vi "TDMS Write Telemtry Data.vi"(8 "error in (no error)":errorcluster, 11 "Iterations":i32) -> (0 "error out":errorcluster, 3 "TDMS file path":path)   [LabVIEW 2021]
doc: "This example demonstrates how to write measured data along with text and timestamp values to a .tdms file using the TDMS API. TDMS files written by this example can be read by the example TDMS Read Events Data.vi."
panel:
  in  "LogEvent":bool
  in  "Stop":bool
  out "Time Stamp":timestamp
  out "Description":string="Event XYZ"
  out "Measured Data":waveform(dbl)[](graph)
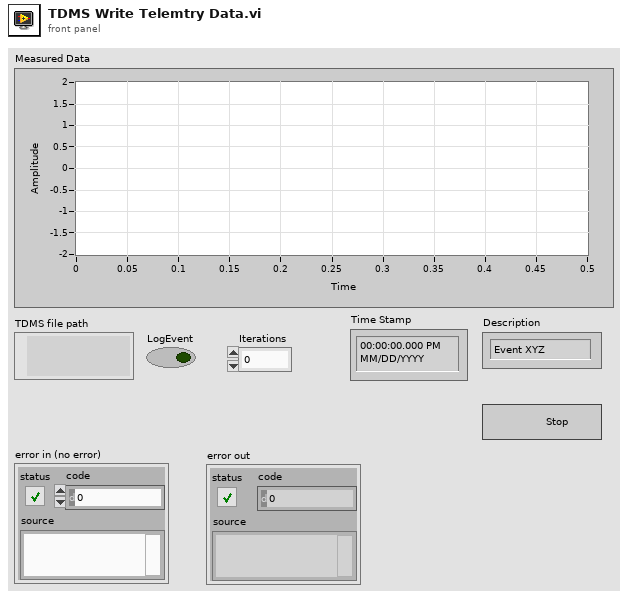
[diagram p1: front panel]
types:
  T1 = enum16{"open", "open or create", "create or replace", "create", "open (read-only)"}
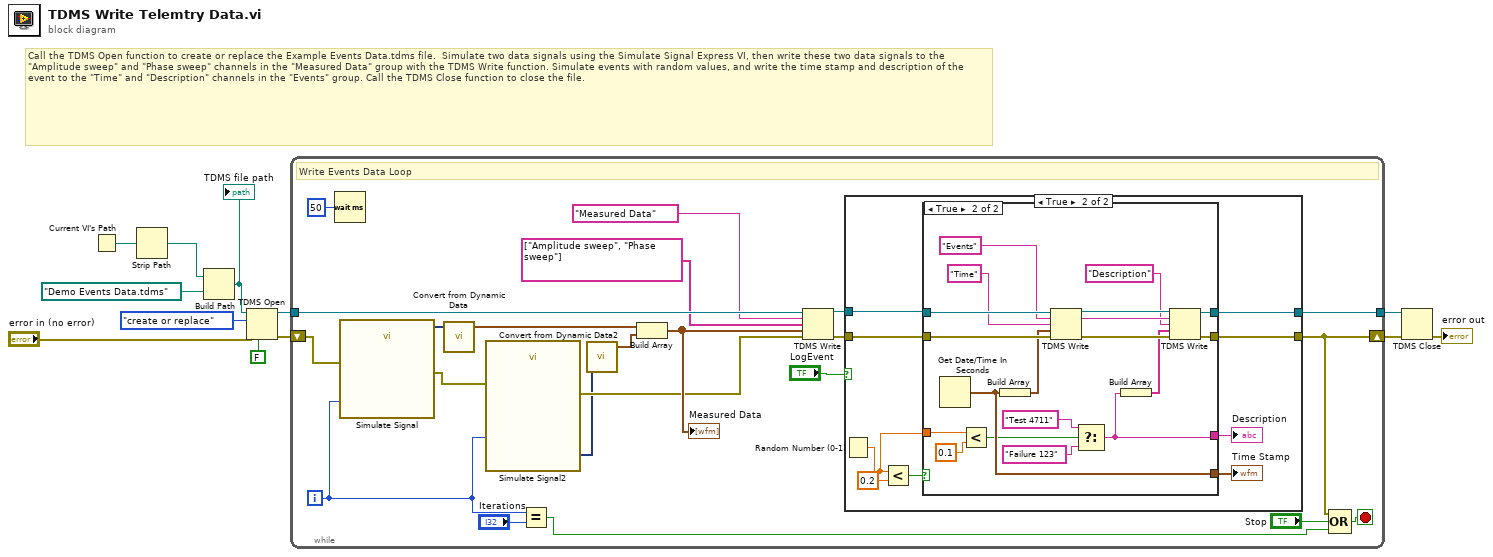
[diagram p0: block diagram]
diagram:
  # "Call the TDMS Open function to create or replace the Example Events Data.tdms file.  Simulate two data signals using the Simulate Signal Express VI, then write these two data signals to the \"Amplitude sweep\" and \"Phase sweep\" channels in the \"Measured Data\" group with the TDMS Write function. Simulate events with random values, and write the time stamp and description of the event to the \"Time\" and \"Description\" channels in the \"Events\" group. Call the TDMS Close function to close the file."
  n1 = Current VI's Path() -> (path=w12:path)
  n2 = Strip Path(path=w12) -> (stripped path=w1:path)  [unwired: 1 out]
  n3 = Build Path(base path=w1, name or relative path=path "Demo Events Data.tdms" ("file path")) -> (appended path=w5:path)
  "TDMS file path" <- w5
  n4 = TDMS Open(6:FALSE ("disable buffering (T)"), 8:"error in (no error)", 10:T1."create or replace" ("operation"), 11:w5) -> (0:w8:errorcluster, 3:w9:refnum<k34>)  [unwired: 3 in]
  n5 = while {
    shift-right: [w30] -> w6
    shift-left: w8 -> [w29]
    tunnel: w9 -> [w24]
    tunnel: [w34] -> w7
    i -> [w13]
    stop <- w31 stop-if-true
    # "Write Events Data Loop"
    n6 = Wait (ms)(milliseconds to wait=u32 50) -> ()  [unwired: 1 out]
    n7 = call "Simulate Signal"("Amplitude"=w13, "error in (no error)"=w29) -> ("Sine"=w28:dynamicdata, "error out"=w27:errorcluster)  [unwired: 12 in]
    n8 = call "Convert from Dynamic Data"("Dynamic Data Type"=w28) -> ("Waveform"=w25:waveform(dbl))  [unwired: 3 in]
    n9 = call "Simulate Signal2"("Phase"=w13, "error in (no error)"=w27) -> ("Sine"=w14:dynamicdata, "error out"=w20:errorcluster)  [unwired: 12 in]
    n10 = Equal?(x=w13, y="Iterations") -> (x = y?=w15:bool)
    n11 = call "Convert from Dynamic Data2"("Dynamic Data Type"=w14) -> ("Waveform"=w26:waveform(dbl))  [unwired: 3 in]
    n12 = Build Array(w25, w26) -> (w21:waveform(dbl)[])
    "Measured Data" <- w21
    n13 = TDMS Write(0:w24, 5:"Measured Data" ("group name"), 7:string[] ["Amplitude sweep", "Phase sweep"] ("channel names"), 9:w21, 11:w20) -> (4:w18:refnum<k34>, 15:w19:errorcluster)  [unwired: 1 in, 2 out]
    n14 = case shown="True" "LogEvent" {
      tunnel: [w36 w44] -> w34
      tunnel: [w35 w42] -> w30
      tunnel: w19 -> [w35 w40]
      tunnel: w18 -> [w36 w39]
      frame False {
      }
      frame True {
        n15 = Random Number (0-1)() -> (number: 0 to 1=w38:dbl)
        n16 = Less?(x=w38, y=0.2) -> (x < y?=w45:bool)
        n17 = case shown="True" w45 {
          tunnel: w40 -> [w46 w65]
          tunnel: [w46 w57] -> w42
          tunnel: [w47 w59] -> w44
          tunnel: w39 -> [w47 w66]
          tunnel: [_ w54] -> w43
          tunnel: w38 -> [_ w53]
          tunnel: [_ w48] -> w41
          frame False {
          }
          frame True {
            n18 = Get Date/Time In Seconds() -> (seconds since 1Jan1904=w54:timestamp)
            n19 = Less?(x=w53, y=0.1) -> (x < y?=w50:bool)
            n20 = Build Array(w54) -> (w62:timestamp[])
            n21 = TDMS Write(0:w66, 5:"Events" ("group name"), 7:"Time" ("channel name"), 9:w62, 11:w65) -> (4:w60:refnum<k34>, 6:w61:string, 15:w58:errorcluster)  [unwired: 1 in, 1 out]
            n22 = Select(t="Test 4711", s=w50, f="Failure 123") -> (s? t:f=w48:string)
            n23 = Build Array(w48) -> (w55:string[])
            n24 = TDMS Write(0:w60, 5:w61, 7:"Description" ("channel name"), 9:w55, 11:w58) -> (4:w59:refnum<k34>, 15:w57:errorcluster)  [unwired: 1 in, 2 out]
          }
        }
        "Description" <- w41
        "Time Stamp" <- w43
      }
    }
    n25 = Compound Arithmetic op=OR(w30, "Stop", w15) -> (w31:bool)
  }
  n26 = TDMS Close(8:w6, 11:w7) -> (0:→"error out":errorcluster)  [unwired: 1 out]
